vi "Teleop_Calc_Pusher.vi"(11 "Teleop Local Data in":T1) -> (3 "Teleop Local Data out":T1)   [LabVIEW 2016]
uses:
  Typedefs/typedef_enum_Joystick Buttons.ctl
  Typedefs/typedef_cluster_Teleop Local Data.ctl
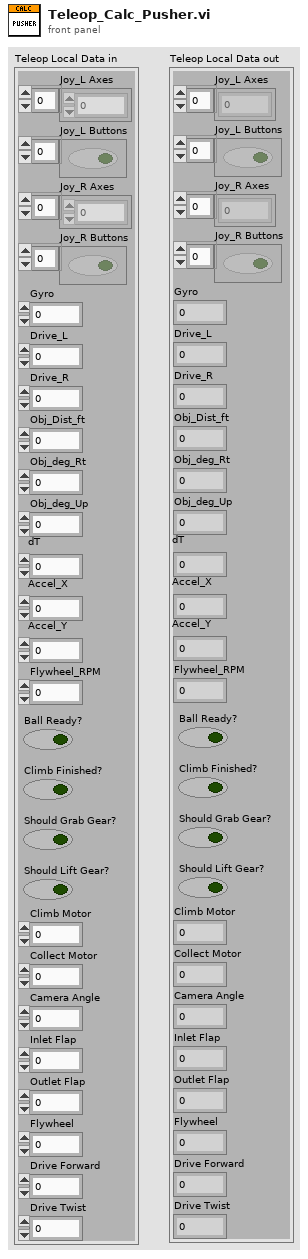
[diagram p1: front panel]
types:
  T1 = typedef "typedef_cluster_Teleop Local Data.ctl" = cluster{"Joy_L Axes":dbl[], "Joy_L Buttons":bool[], "Joy_R Axes":dbl[], "Joy_R Buttons":bool[], "Gyro":dbl, "Drive_L":i32, "Drive_R":i32, "Obj_Dist_ft":dbl, "Obj_deg_Rt":dbl, "Obj_deg_Up":dbl, "dT":dbl, "Accel_X":dbl, "Accel_Y":dbl, "Flywheel_RPM":dbl, "Ball Ready?":bool, "Climb Finished?":bool, "Should Grab Gear?":bool, "Should Lift Gear?":bool, "Climb Motor":dbl, "Collect Motor":dbl, "Camera Angle":dbl, "Inlet Flap":dbl, "Outlet Flap":dbl, "Flywheel":dbl, "Drive Forward":dbl, "Drive Twist":dbl}
  T2 = typedef "typedef_enum_Joystick Buttons.ctl" = enum16{"Trigger", "Thumb", "Top3", "Top4", "Top5", "Top6", "Low7", "Low8", "Low9", "Low10", "Low11", "Low12", "Hat0", "Hat1", "Hat2", "Hat3", "Hat4", "Hat5", "Hat6", "Hat7", "Hat8"}
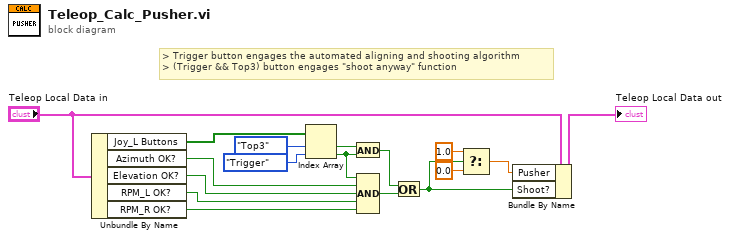
[diagram p0: block diagram]
diagram:
  # "> Trigger button engages the automated aligning and shooting algorithm\n> (Trigger && Top3) button engages \"shoot anyway\" function"
  n1 = Unbundle By Name("Teleop Local Data in") -> ("Joy_L Buttons"=w15:bool[], "Azimuth OK?"=w10:bool, "Elevation OK?"=w11:bool, "RPM_L OK?"=w12:bool, "RPM_R OK?"=w13:bool)
  n2 = Index Array(array=w15, index #1=typedef_enum_Joystick_Buttons."Top3" ("Joystick Buttons"), index #2=typedef_enum_Joystick_Buttons."Trigger" ("Joystick Buttons")) -> (element #1=w2:bool, element #2=w1:bool)
  n3 = And(x=w2, y=w1) -> (x .and. y?=w3:bool)
  n4 = Compound Arithmetic op=AND(w1, w10, w11, w12, w13) -> (w9:bool)
  n5 = Or(x=w3, y=w9) -> (x .or. y?=w4:bool)
  n6 = Select(t=1.0, s=w4, f=0.0 ("V_X")) -> (s? t:f=w6:dbl)
  n7 = Bundle By Name(cluster="Teleop Local Data in", "Pusher"=w6, "Shoot?"=w4) -> (→"Teleop Local Data out":T1)
